vi "template.vi"() -> ()   [LabVIEW 2020]
uses:
  <vilib>/Platform/TimedLoop/XDataNode/timing_clust.ctl
  <vilib>/Platform/TimedLoop/XDataNode/nitl_modes.ctl
  <vilib>/Platform/TimedLoop/XDataNode/wakeup.ctl
  <extravilib>/ChannelInstances/Stream-bool/Write With Abort.vi
  <extravilib>/ChannelInstances/Stream-bool/Read With Abort.vi
  <extravilib>/ChannelInstances/Stream-bool/Endpoint.vi
  <extravilib>/ChannelInstances/Stream-bool/EndpointRead.vi
  <extravilib>/ChannelInstances/Stream-bool/Instantiate.vi
  <extravilib>/ChannelInstances/Stream-bool/)Channel.vi
  <resource>/ChannelSupport/_ChannelSupport/WaitIfNeeded.vi
  <vilib>/platform/TimedLoop/XDataNode/XDataNode.xnode
  <vilib>/Platform/TimedLoop/XDataNode/XDNodeRunTimeDep.lvlib
  <extravilib>/ChannelInstances/Stream-bool.lvlib
panel:
  out "error out":errorcluster
  out "GPS data out":string
  in  "Stop 8082":bool
  in  "Stop":bool
  out "Arm System":bool
  in  "Start":bool
  out "Laser 2":bool
  out "Laser 1":bool
  in  "Speed Threshold (km/h)":dbl
  out "Safety System 2":bool[](array[boolean])
  out "Safety System 1":bool[](array[boolean])
  out "GPS":cluster{"Lat":dbl, "Lon":dbl, "Speed":dbl}
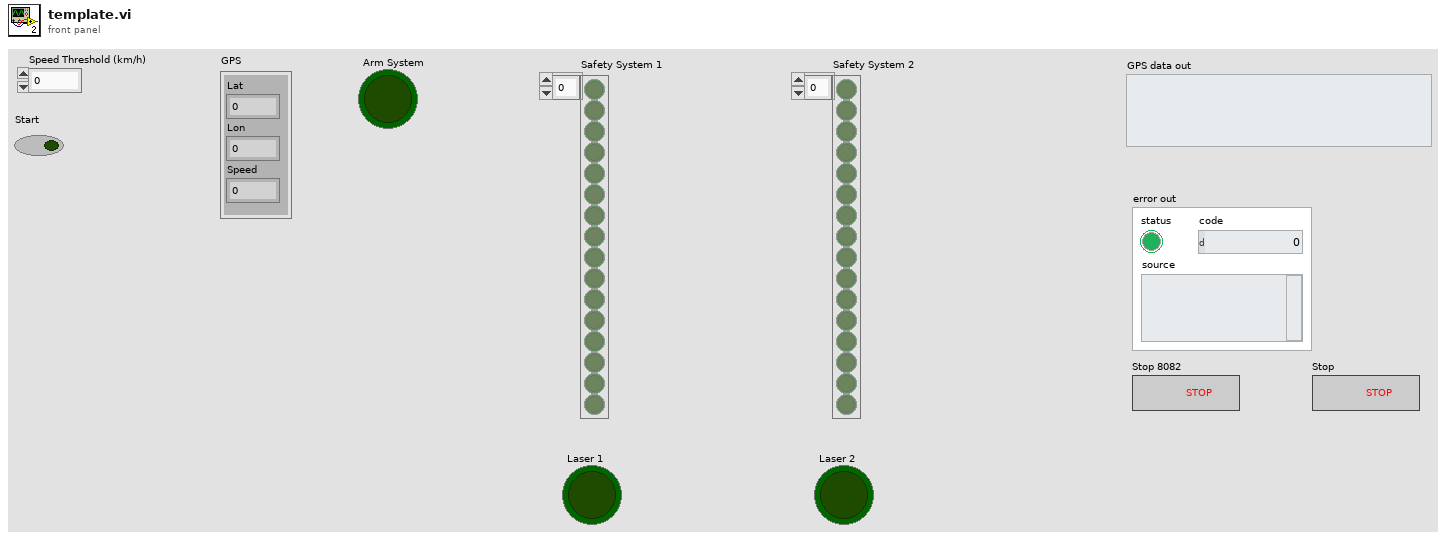
[diagram p1: front panel]
types:
  T1 = enum8{"Enabled", "Disabled", "Disabled and Grayed Out"}
  T2 = typedef "XDNodeRunTimeDep.lvlib/timing_clust.ctl" = cluster{"Expected End [f-1]":u64, "Actual End [f-1]":u64, "Finished Late? [f-1]":bool, "Expected End [i-1]":u64, "Actual End [i-1]":u64, "Finished Late? [i-1]":bool, "Expected Start [i]":u64, "Actual Start [i]":u64, "Expected Start [f]":u64, "Actual Start [f]":u64, "Source Name":string, "Structure Name":string, "Period":i64, "Deadline":i64, "Offset":i64, "Start":i64, "Priority":i32, "Timeout":i32, "Mode":T3, "Wakeup Reason":T4, "Error":errorcluster, "Source Type":string, "Secondary Source Type":string, "Global End Time":u64, "Global Start Time":u64, "Frame Duration":u64, "Iteration Duration":u64, "Assigned CPU":i32, "I/O Scan Engine Mode":u32}
  T3 = typedef "XDNodeRunTimeDep.lvlib/nitl_modes.ctl" = enum32{"No Change", "Process missed periods, maintain original phase", "Discard missed periods, maintain original phase", "Process missed periods, ignore original phase", "Discard missed periods, ignore original phase"}
  T4 = typedef "XDNodeRunTimeDep.lvlib/wakeup.ctl" = enum32{"Normal", "Aborted", "Asynchronous wakeup", "Timing source error", "Timed loop error", "Timeout"}
  T5 = enum16{"Standard", "Buffered", "CRLF", "Immediate"}
  T6 = typedef "Stream-bool.lvlib/)Channel.ctl" = refnum<queue>
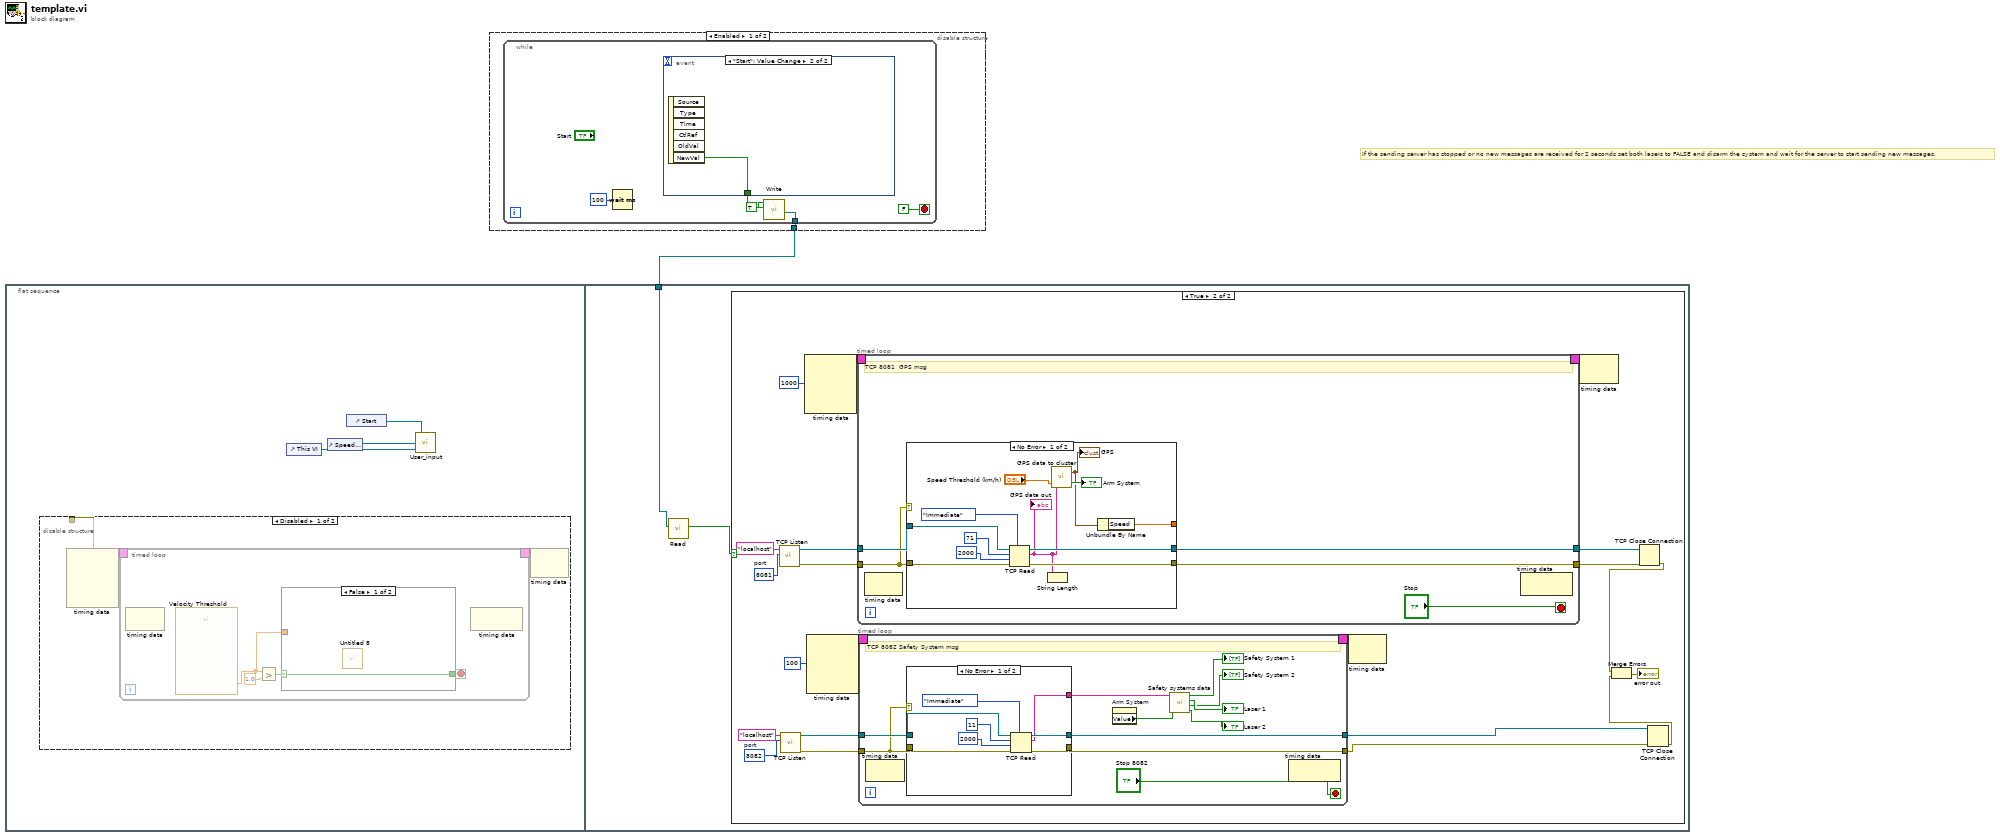
[diagram p0: block diagram]
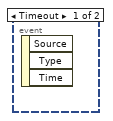
[diagram p2: hidden frame]
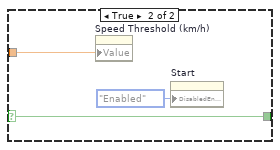
[diagram p4: hidden frame]
diagram:
  # "If the sending server has stopped or no new messages are received for 2 seconds set both lasers to FALSE and disarm the system and wait for the server to start sending new messages."
  n1 = flat-sequence {
    tunnel: w1 -> [w22]
    frame #0 {
      n2 = disable-structure shown="Disabled" {
        disable-tunnel: _ -> [w5 _]
        frame Disabled {
          n3 = node-c288(w5) -> (w7:T2)  [unwired: 3 in]
          n4 = timed-loop {
            timing: w7 -> [_]
            timing-out: [_] -> w6
            stop <- w9 stop-if-true
            n5 = node-c288() -> ()  [unwired: 1 in, 1 out]
            n6 = call "Velocity Threshold"() -> ("velocity"=w8:dbl)  [unwired: 17 in, 2 out]
            n7 = Greater?(x=w8, y=1.0) -> (0:w10:bool)
            n8 = case shown="False" w10 {
              selector: w10 -> [w12 w15]
              tunnel: [w12 w15] -> w9
              tunnel: w8 -> [_ w13]
              frame False {
                n9 = call "Untitled 8.vi"() -> ()  [unwired: 10 in, 2 out]
              }
              frame True {
                n10 = property on="Speed Threshold (km/h)" class="DigNum (strict)"("Value"=w13) -> ()  [unwired: 2 in, 2 out]
                n11 = property on="Start" class="Bool (strict)"("DisabledEnum"=T1."Enabled" ("Disabled")) -> ()  [unwired: 2 in, 2 out]
              }
            }
            n12 = node-c288() -> ()  [unwired: 1 in, 1 out]
          }
          n13 = node-c288(w6) -> ()  [unwired: 1 out]
        }
        frame Enabled {
        }
      }
      n14 = control-ref of="This VI"() -> (w2:refnum<vi>)
      n15 = control-ref of="Speed Threshold (km/h)"() -> (w3:refnum<vi>)
      n16 = control-ref of="Start"() -> (w4:refnum<vi>)
      n17 = call "User_input.vi"("Main Vi"=w2, "Speed Threshold (km/h) Ref"=w3, "Start Ref"=w4) -> ()  [unwired: 1 in]
    }
    frame #1 {
      n18 = call <extravilib>:"Read.vi"("channel"=w22) -> ("element"=w23:bool)  [unwired: 6 in, 4 out]
      n19 = case shown="True" w23 {
        frame False {
        }
        frame True {
          w34 = u16 8082  # port
          w40 = u16 8081  # port
          n20 = call <vilib>:"TCP Listen.vi"("port"=w40, "service name"="localhost") -> ("error out"=w38:errorcluster, "connection ID"=w31:refnum<k5>)  [unwired: 5 in, 3 out]
          n21 = call <vilib>:"TCP Listen.vi"("port"=w34, "service name"="localhost") -> ("error out"=w36:errorcluster, "connection ID"=w37:refnum<k5>)  [unwired: 5 in, 3 out]
          n22 = node-c288(i64 1000 ("Period")) -> (w44:T2)  [unwired: 3 in]
          n23 = node-c288(i64 100 ("Period")) -> (w42:T2)  [unwired: 3 in]
          n24 = timed-loop {
            tunnel: w38 -> [w73]
            tunnel: w31 -> [w76]
            tunnel: [w75] -> w30
            tunnel: [w74] -> w29
            timing: w44 -> [_]
            timing-out: [_] -> w43
            stop <- "Stop" stop-if-true
            # "TCP 8081  GPS msg"
            n25 = node-c288() -> ()  [unwired: 1 in, 1 out]
            n26 = case shown="No Error" w73 {
              tunnel: w73 -> [w85 w90]
              tunnel: w76 -> [w84 w89]
              tunnel: [w83 w90] -> w75
              tunnel: [w82 w89] -> w74
              tunnel: [w78 _] -> _
              frame No Error {
                n27 = TCP Read(connection ID=w84, bytes to read=71, error in (no error)=w85, 7:T5."Immediate" ("mode (standard)"), 9:2000 ("timeout ms (25000)")) -> (connection ID out=w82:refnum<k5>, data out=w77:string, error out=w83:errorcluster)
                "GPS data out" <- w77
                n28 = String Length(string=w77) -> ()  [unwired: 1 out]
                n29 = call "GPS data to cluster.vi"("Speed Threshold (km/h)"="Speed Threshold (km/h)", "Gps raw data in"=w77) -> ("Arm System?"=→"Arm System":bool, "GPS Cluster"=w79:cluster{"Lat":dbl, "Lon":dbl, "Speed":dbl})
                "GPS" <- w79
                n30 = Unbundle By Name(w79) -> ("Speed"=w78:dbl)
              }
              frame Error {
              }
            }
            n31 = node-c288() -> ()  [unwired: 1 in, 1 out]
          }
          n32 = timed-loop {
            tunnel: w36 -> [w45]
            tunnel: w37 -> [w55]
            tunnel: [w54] -> w28
            tunnel: [w53] -> w27
            timing: w42 -> [_]
            timing-out: [_] -> w41
            stop <- "Stop 8082" stop-if-true
            # "TCP 8082 Safety System msg"
            n33 = node-c288() -> ()  [unwired: 1 in, 1 out]
            n34 = case shown="No Error" w45 {
              tunnel: w45 -> [w60 w65]
              tunnel: w55 -> [w59 w64]
              tunnel: [w58 w65] -> w54
              tunnel: [w57 w64] -> w53
              tunnel: [w56 _] -> w52
              frame No Error {
                n35 = TCP Read(connection ID=w59, bytes to read=11, error in (no error)=w60, 7:T5."Immediate" ("mode (standard)"), 9:2000 ("timeout ms (25000)")) -> (connection ID out=w57:refnum<k5>, data out=w56:string, error out=w58:errorcluster)
              }
              frame Error {
              }
            }
            n36 = property on="Arm System" class="Bool (strict)"() -> ("Value"=w47:bool)  [unwired: 2 in, 2 out]
            n37 = call "Safety systems data.vi"("Arm System Status"=w47, "safety system raw data"=w52) -> ("Laser 2"=→"Laser 2":bool, "Safety System 2"=→"Safety System 2":bool[], "Laser 1"=→"Laser 1":bool, "Safety System 1"=→"Safety System 1":bool[])  [unwired: 3 in]
            n38 = node-c288() -> ()  [unwired: 1 in, 1 out]
          }
          n39 = node-c288(w41) -> ()  [unwired: 1 out]
          n40 = node-c288(w43) -> ()  [unwired: 1 out]
          n41 = TCP Close Connection(connection ID=w29, error in (no error)=w30) -> (error out=w25:errorcluster)  [unwired: 1 in, 1 out]
          n42 = TCP Close Connection(connection ID=w27, error in (no error)=w28) -> (error out=w24:errorcluster)  [unwired: 1 in, 1 out]
          n43 = Merge Errors(w25, w24) -> (→"error out":errorcluster)
        }
      }
    }
  }
  n44 = disable-structure shown="Enabled" {
    disable-tunnel: [w97 _] -> w1
    frame Enabled {
      n45 = while {
        tunnel: [w98] -> w97
        stop <- FALSE stop-if-true
        n46 = Wait (ms)(milliseconds to wait=u32 100) -> ()  [unwired: 1 out]
        n47 = event shown="[1] \"Start\": Value Change" {
          selector: _ -> [_ _]
          dyn-events: _ -> [_ _]
          timeout: _ -> [_ _]
          tunnel: [_ w103] -> w100
          event Timeout {
            n48 = event-data() -> ()  [unwired: 1 in, 3 out]
          }
          event "Start": Value Change {
            n49 = event-data() -> ("NewVal"=w103:bool)  [unwired: 1 in, 5 out]
          }
        }
        n50 = call <extravilib>:"Write.vi"("element"=w100, "element valid? (T)"=TRUE) -> ("channel"=w98:T6)  [unwired: 7 in, 2 out]
      }
    }
    frame Disabled {
    }
  }
